vi "Do Request.vi"(7 "Processing In":refnum<class "Processing.lvclass">, 11 "HardwareHTTPController in":refnum<class "HardwareHTTPController.lvclass">) -> (0 "error out":errorcluster, 5 "Processing":refnum<class "Processing.lvclass">)   [LabVIEW 2023, in "Volatus.lvlib" / "HardwareHTTPController.lvclass"]
doc: "A controller's main job is to respond to a request by generating a response. The response value must be specified by calling Set Response.vi on the Processing class that's passed through the VI otherwise an error will be generated.\n\nThere are several helpers available for common response types:\nGenerating HTML content programmatically - Create Basic Response.vi\nStreaming a file from disk - Create File Response.vi\nRedirecting the user to another URL - Create Redirect Response.vi\n\nFile responses are streamed in chunks and do not load the entire file into memory at once to send in the response which allows serving large files more efficiently."
uses:
  HardwareHTTPController.lvclass
  lv-http-server/HTTP Server/Processing/Processing.lvclass
  lv-http-server/HTTP Server/Processing/Processing.lvclass/Processing.ctl
  lv-http-util/HTTP Utils/Request/Request.lvclass/Request.ctl
  lv-uri/URI/URI/URI.lvclass/URI.ctl
  lv-http-util/HTTP Utils/Request/Get Target URI.vi
  lv-uri/URI/URI/Path String.vi
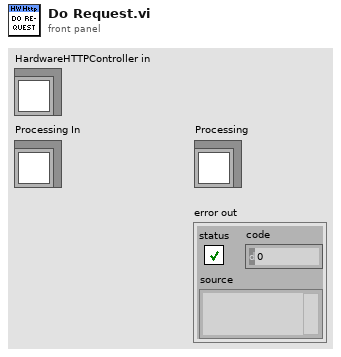
[diagram p1: front panel]
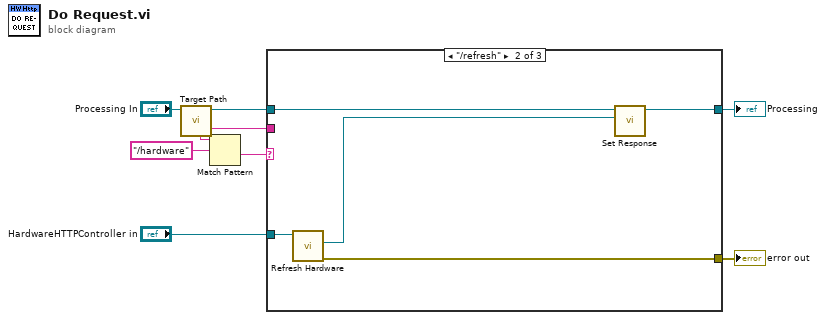
[diagram p0: block diagram]
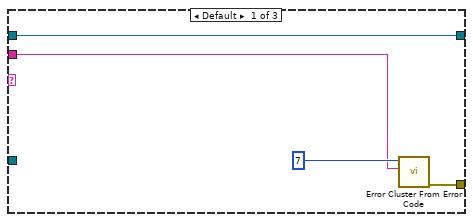
[diagram p2: hidden frame]
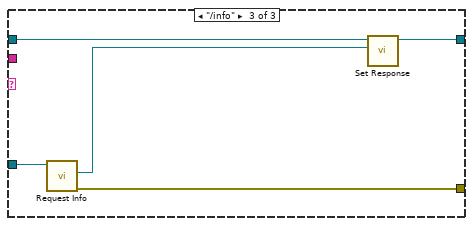
[diagram p3: hidden frame]
diagram:
  n1 = call "Target Path.vi"("Processing in"="Processing In") -> ("Processing out"=w6:refnum<class "Processing.lvclass">, "Target Path"=w3:string)  [unwired: 9 in]
  n2 = Match Pattern(string=w3, regular expression="/hardware") -> (after substring=w5:string)  [unwired: 1 in, 3 out]
  n3 = case shown="\"/refresh\"" w5 {
    tunnel: w6 -> [w9 w17 w22]
    tunnel: [w12 w13 w19] -> w4
    tunnel: w3 -> [w10 _ _]
    tunnel: [w9 w16 w21] -> w2
    tunnel: "HardwareHTTPController in" -> [_ w15 w20]
    frame Default {
      n4 = call <vilib>:"Error Cluster From Error Code.vi"("error message (\"\")"=w10, "error code (0)"=7) -> ("error out"=w12:errorcluster)  [unwired: 7 in]
    }
    frame "/refresh" {
      n5 = call "Refresh Hardware.vi"("HardwareHTTPController in"=w15) -> ("error out"=w13:errorcluster, "Response"=w14:refnum<class "Response.lvclass">)  [unwired: 8 in, 1 out]
      n6 = call "Set Response.vi"("Response"=w14, "Processing in"=w17) -> ("Processing out"=w16:refnum<class "Processing.lvclass">)  [unwired: 9 in]
    }
    frame "/info" {
      n7 = call "Request Info.vi"("HardwareHTTPController in"=w20) -> ("error out"=w19:errorcluster, "Response"=w18:refnum<class "Response.lvclass">)  [unwired: 8 in, 1 out]
      n8 = call "Set Response.vi"("Response"=w18, "Processing in"=w22) -> ("Processing out"=w21:refnum<class "Processing.lvclass">)  [unwired: 9 in]
    }
  }
  "error out" <- w4
  "Processing" <- w2
